vi "DDMs_low_terminate.vi"(8 "error in (no error)":errorcluster, 10 "Device":enum16{"Agilent34401A", "ADCMT7351", "HP3478A"}(ring), 11 "VISA resource name":refnum<visa-resource-name>) -> (0 "error out":errorcluster)   [LabVIEW 2017, in "DMMsData.lvclass"]
uses:
  DMMsData.lvclass
  istr.lib/ADCMT7351_ADC/ADCMT7351_ADC.lvlib
  <instrlib>/Agilent 34401/Agilent 34401.lvlib
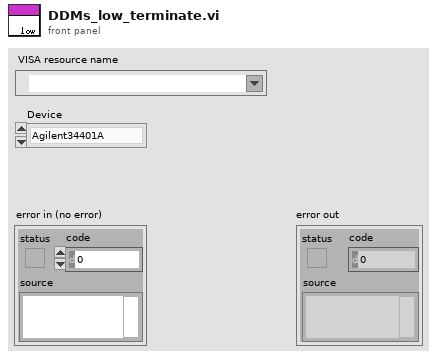
[diagram p1: front panel]
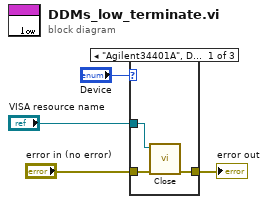
[diagram p0: block diagram]
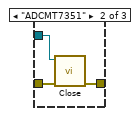
[diagram p2: hidden frame]
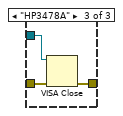
[diagram p3: hidden frame]
diagram:
  n1 = case shown="\"Agilent34401A\", Default" "Device" {
    tunnel: "VISA resource name" -> [w7 w10 w12]
    tunnel: "error in (no error)" -> [w6 w9 w13]
    tunnel: [w5 w8 w11] -> w1
    frame "Agilent34401A", Default {
      n2 = call <instrlib>:"Close.vi"("error in (no error)"=w6, "VISA resource name"=w7) -> ("error out"=w5:errorcluster)  [unwired: 9 in]
    }
    frame "ADCMT7351" {
      n3 = call <instrlib>:"Close.vi"("error in (no error)"=w9, "VISA resource name"=w10) -> ("error out"=w8:errorcluster)  [unwired: 9 in]
    }
    frame "HP3478A" {
      n4 = VISA Close(VISA resource name=w12, error in (no error)=w13) -> (error out=w11:errorcluster)
    }
  }
  "error out" <- w1
